vi "MyMethod1.vi"(0 "reference in":refnum<class "AnotherClass.lvclass">, 5 "error in (no error)":errorcluster) -> (14 "reference out":refnum<class "AnotherClass.lvclass">, 19 "error out":errorcluster)   [LabVIEW 2020, in "AnotherClass.lvclass"]
uses:
  AnotherClass.lvclass
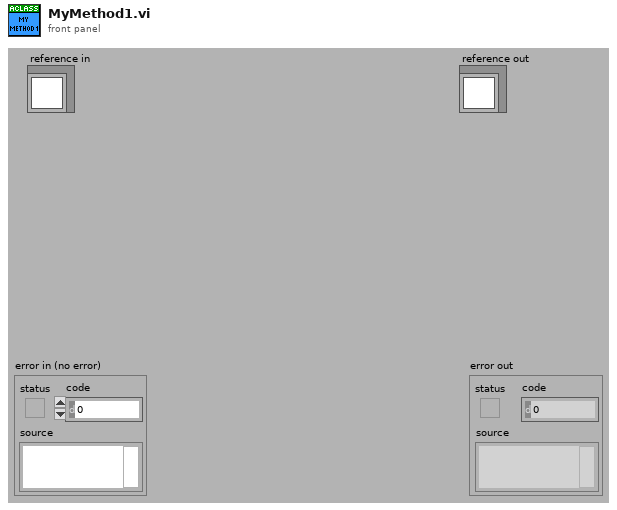
[diagram p1: front panel]
types:
  T1 = typedef "AnotherClass.lvclass/ObjectAttributes.ctl" = cluster{"Attribute1":dbl}
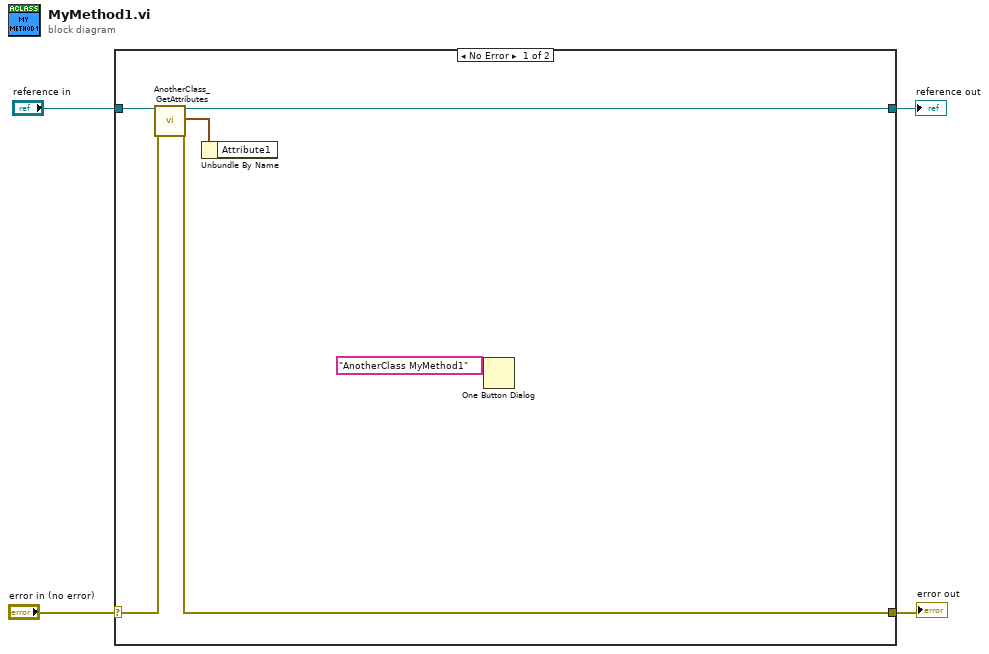
[diagram p0: block diagram]
diagram:
  n1 = case shown="No Error" "error in (no error)" {
    selector: "error in (no error)" -> [w10 w12]
    tunnel: [w8 w12] -> w3
    tunnel: [w6 w11] -> w1
    tunnel: "reference in" -> [w7 w11]
    frame No Error {
      n2 = call "AnotherClass_GetAttributes.vi"("reference in"=w7, "error in (no error)"=w10) -> ("reference out"=w6:refnum<class "AnotherClass.lvclass">, "attributes"=w9:T1, "error out"=w8:errorcluster)  [unwired: 1 in, 14 out]
      n3 = Unbundle By Name(w9) -> ()  [unwired: 1 out]
      n4 = One Button Dialog(message="AnotherClass MyMethod1") -> ()  [unwired: 2 out]
    }
    frame Error {
    }
  }
  "error out" <- w3
  "reference out" <- w1
